vi "Not_Test_Mode.vi"() -> (3 "NOT TEST MODE":bool)   [LabVIEW 2019]
uses:
  Robot Global Data.vi
  <vilib>/Rock Robotics/WPI/DriverStation/WPI_DriverStationRobotMode2.ctl
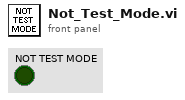
[diagram p1: front panel]
types:
  T1 = typedef "WPI_DriverStationRobotMode2.ctl" = enum16{"Autonomous Disabled", "Autonomous Enabled", "Teleop Disabled", "Teleop Enabled", "Disconnected", "Finish", "Test Disabled", "Test Enabled", "Emergency Stopped"}
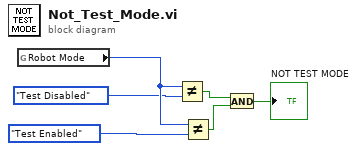
[diagram p0: block diagram]
diagram:
  n1 = global read "Robot Global Data.vi" "Robot Mode"() -> (w3:T1)
  n2 = Not Equal?(x=w3, y=WPI_DriverStationRobotMode2."Test Disabled") -> (x != y?=w5:bool)
  n3 = Not Equal?(x=w3, y=WPI_DriverStationRobotMode2."Test Enabled") -> (x != y?=w6:bool)
  n4 = And(x=w5, y=w6) -> (x .and. y?=→"NOT TEST MODE":bool)
